vi "ad get sample layout.vi"(8 "error in (no error)":errorcluster, 9 "layout":T1, 10 "index":i32, 11 "adh":i32) -> (0 "error out":errorcluster, 1 "layout out":T1, 3 "function return":i32)   [LabVIEW 2021, in "libad4.lvlib"]
doc: "LIBAD4 function: ad_get_sample_layout (int32_t adh, int32_t index, struct ad_sample_layout *layout);\n\nReads samples layout information. Requires AD_SF_SAMPLES flag to be set."
uses:
  <userlib>/libad4/libad4.lvlib
  <userlib>/libad4/controls/ad sample layout.ctl
  <userlib>/libad4/libad4.dll
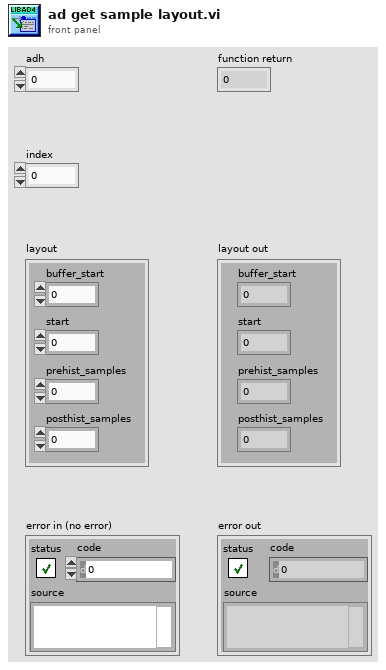
[diagram p1: front panel]
types:
  T1 = typedef "libad4.lvlib/ad sample layout.ctl" = cluster{"buffer_start":u64, "start":u64, "prehist_samples":u64, "posthist_samples":u64}
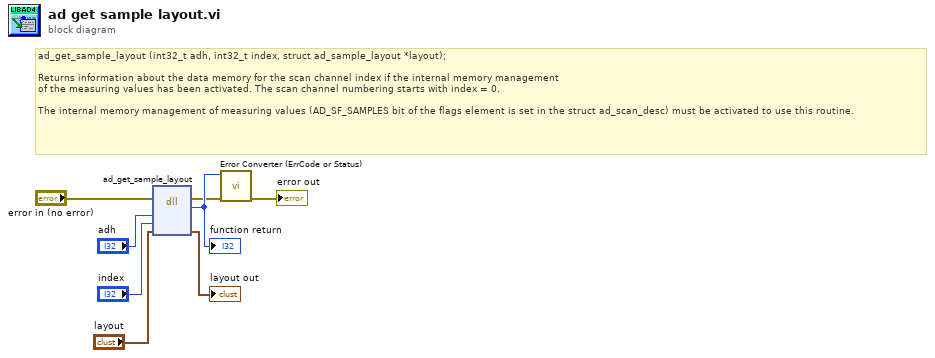
[diagram p0: block diagram]
diagram:
  # "ad_get_sample_layout (int32_t adh, int32_t index, struct ad_sample_layout *layout);\n\nReturns information about the data memory for the scan channel index if the internal memory management \nof the measuring values has been activated. The scan channel numbering starts with index = 0.\n\nThe internal memory management of measuring values (AD_SF_SAMPLES bit of the flags element is set in the struct ad_scan_desc) must be activated to use this routine."
  n1 = dll-call lib="C:/Program Files/National Instruments/LabVIEW 2021/user.lib/libad4/libad4.*" fn="ad_get_sample_layout"(error in="error in (no error)", "adh"="adh", "index"="index", "layout"="layout") -> (error out=w2:errorcluster, w8:i32, "layout"=→"layout out":T1)  [unwired: 4 in, 1 out]
  "function return" <- w8
  n2 = call <userlib>:"Error Converter (ErrCode or Status).vi"("error in (no error)"=w2, "error code"=w8) -> ("error out"=→"error out":errorcluster)  [unwired: 9 in]
